vi "Update Git Info.vi"(8 "error in (no error)":errorcluster, 11 "Git Updater Module in":refnum<class "Git Updater Module.lvclass">) -> (0 "error out":errorcluster, 2 "Git Info":T1, 3 "Git Updater Module out":refnum<class "Git Updater Module.lvclass">)   [LabVIEW 2020, in "Volatus.lvlib" / "Git Updater Module.lvclass"]
uses:
  Git Updater Module.lvclass
  Git Updater Module.lvclass/Git Updater Module.ctl
  Module/Module.lvclass
  VolatusAPI/VolatusAPI.lvclass
  <vilib>/Hampel Software Engineering/Git API/Git API/GIT-api.lvclass
  Git Info.ctl
  C:/dev/lv20CE/relink/lv-volatus/Volatus/Module/Module.lvclass
  C:/dev/lv20CE/relink/lv-volatus/Volatus/Git Updater Module/Git Updater Module.lvclass
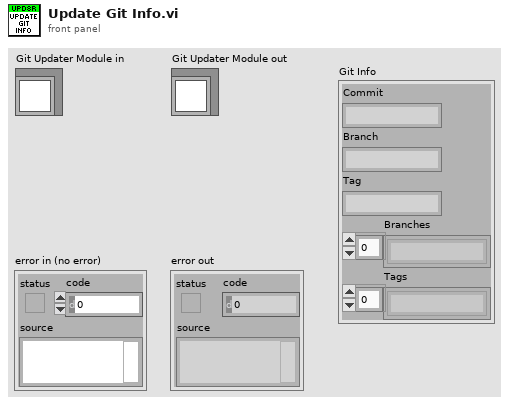
[diagram p1: front panel]
types:
  T1 = typedef "Volatus.lvlib/Git Updater Module.lvclass/Git Info.ctl" = cluster{"Commit":string, "Branch":string, "Tag":string, "Branches":string[], "Tags":string[]}
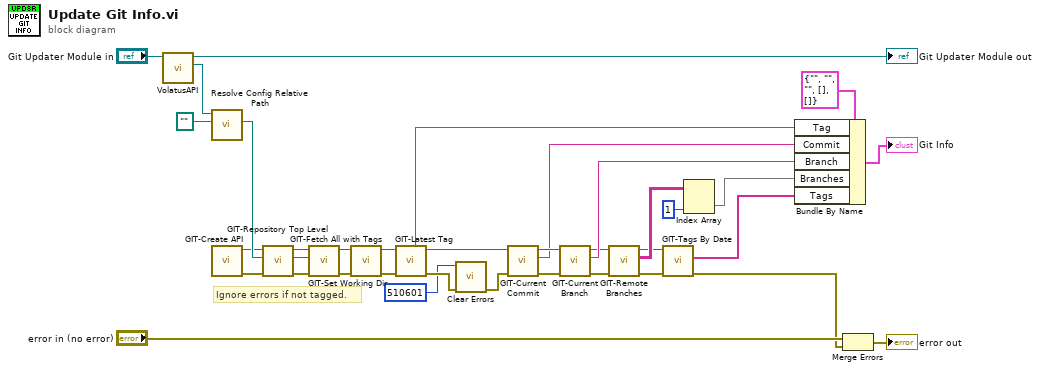
[diagram p0: block diagram]
diagram:
  # "Ignore errors if not tagged."
  n1 = call "VolatusAPI.vi"("Module in"="Git Updater Module in") -> ("VolatusAPI"=w33:refnum<class "VolatusAPI.lvclass">, "Module out"=→"Git Updater Module out":refnum<class "Git Updater Module.lvclass">)  [unwired: 9 in]
  n2 = call "Resolve Config Relative Path.vi"("Path"=path "", "VolatusAPI in"=w33) -> ("Resolved Path"=w31:path)  [unwired: 7 in, 2 out]
  n3 = call <vilib>:"GIT-Create API.vi"() -> ("error out"=w29:errorcluster, "git-api out"=w30:refnum<class "GIT-api.lvclass">)  [unwired: 10 in]
  n4 = call <vilib>:"GIT-Repository Top Level.vi"("error in"=w29, "Current Path"=w31, "git-api in"=w30) -> ("error out"=w26:errorcluster, "Repo Top Level Path"=w27:path, "git-api out"=w28:refnum<class "GIT-api.lvclass">)  [unwired: 6 in]
  n5 = call <vilib>:"GIT-Set Working Dir.vi"("error in"=w26, "Working Directory"=w27, "git-api in"=w28) -> ("error out"=w25:errorcluster, "git-api out"=w4:refnum<class "GIT-api.lvclass">)  [unwired: 7 in]
  n6 = call <vilib>:"GIT-Fetch All with Tags.vi"("error in"=w25, "Git-API in"=w4) -> ("error out"=w5:errorcluster, "Git-API out"=w3:refnum<class "GIT-api.lvclass">)  [unwired: 8 in]
  n7 = call <vilib>:"GIT-Latest Tag.vi"("error in"=w5, "git-api in"=w3) -> ("error out"=w21:errorcluster, "git-api out"=w24:refnum<class "GIT-api.lvclass">, "Latest Tag"=w17:string)  [unwired: 6 in, 1 out]
  n8 = call <vilib>:"Clear Errors.vi"("error in (no error)"=w21, "specific error code to clear (0: all)"=510601) -> ("error out"=w20:errorcluster)  [unwired: 4 in, 1 out]
  n9 = call <vilib>:"GIT-Current Commit.vi"("error in"=w20, "git-api in"=w24) -> ("error out"=w22:errorcluster, "current commit"=w16:string, "git-api out"=w23:refnum<class "GIT-api.lvclass">)  [unwired: 7 in]
  n10 = call <vilib>:"GIT-Current Branch.vi"("error in"=w22, "git-api in"=w23) -> ("error out"=w12:errorcluster, "current branch"=w15:string, "git-api out"=w11:refnum<class "GIT-api.lvclass">)  [unwired: 6 in, 1 out]
  n11 = call <vilib>:"GIT-Remote Branches.vi"("error in"=w12, "git-api in"=w11) -> ("error out"=w7:errorcluster, "branches"=w10:string[][], "git-api out"=w6:refnum<class "GIT-api.lvclass">)  [unwired: 7 in]
  n12 = call <vilib>:"GIT-Tags By Date.vi"("error in"=w7, "Git-API in"=w6) -> ("error out"=w1:errorcluster, "tags"=w2:string[])  [unwired: 7 in, 1 out]
  n13 = Index Array(array=w10, index (col)=1 ("disabled index (col)")) -> (element=w8:string[])  [unwired: 1 in]
  n14 = Bundle By Name(cluster=T1 {"Commit"="", "Branch"="", "Tag"="", "Branches"=[], "Tags"=[]} ("Git Info"), "Tag"=w17, "Commit"=w16, "Branch"=w15, "Branches"=w8, "Tags"=w2) -> (→"Git Info":T1)
  n15 = Merge Errors("error in (no error)", w1) -> (→"error out":errorcluster)
